vi "Insert LVClass Property Node - Tests.vi"(8 "error in (no error)":errorcluster) -> (0 "error out":errorcluster)   [LabVIEW 2017]
uses:
  myChildClass/myChildClass.lvclass
  myOtherClass.lvclass
  0cfaee32-47ef-4325-a365-739cce7879ef.vi
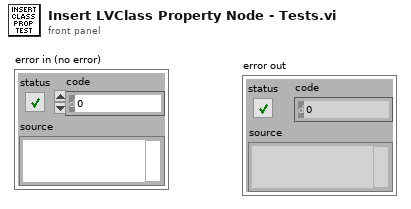
[diagram p1: front panel]
types:
  T1 = enum16{"Right Mouse Down", "Right Mouse Up", "Middle Mouse Down", "Middle Mouse Up", "Left Mouse Down", "Left Mouse Up"}
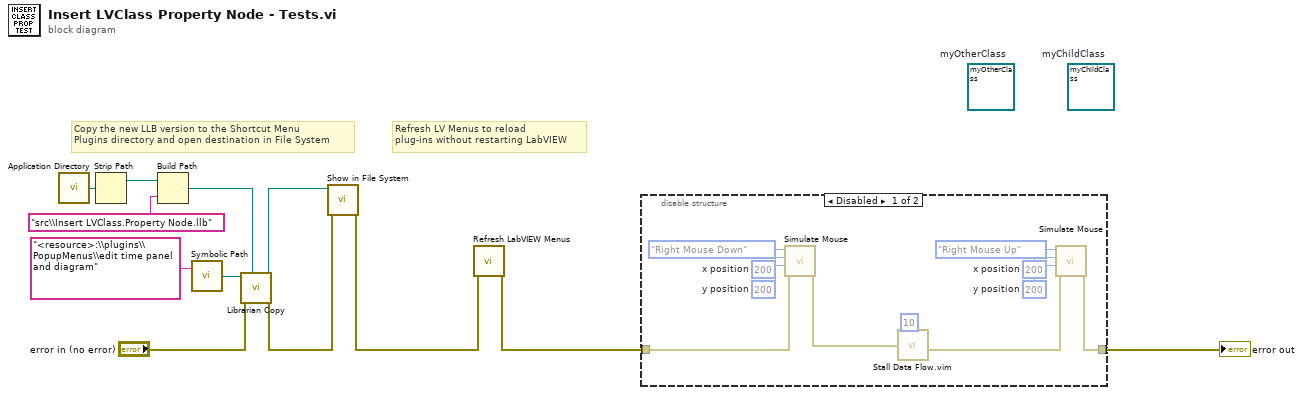
[diagram p0: block diagram]
diagram:
  (unwired) refnum<class "myOtherClass.lvclass"> refnum  # myOtherClass
  (unwired) refnum<class "myChildClass.lvclass"> refnum  # myChildClass
  # "Refresh LV Menus to reload \nplug-ins without restarting LabVIEW"
  # "Copy the new LLB version to the Shortcut Menu \nPlugins directory and open destination in File System"
  n1 = call <vilib>:"Application Directory.vi"() -> ("Application Directory"=w12:path)
  n2 = Strip Path(path=w12) -> (stripped path=w11:path)  [unwired: 1 out]
  n3 = Build Path(base path=w11, name or relative path="src\\Insert LVClass.Property Node.llb") -> (appended path=w9:path)
  n4 = call "Symbolic Path.vi"("Symbolic Path"="<resource>:\\plugins\\PopupMenus\\edit time panel and diagram" ("name or relative path")) -> ("ActualPath"=w1:path)  [unwired: 1 in]
  n5 = call <vilib>:"Librarian Copy.vi"("source"=w9, "error in (no error)"="error in (no error)", "destination"=w1) -> ("error out"=w7:errorcluster, "dup destination"=w8:path)  [unwired: 7 in]
  n6 = call <vilib>:"Show in File System.vi"("error in (no error)"=w7, "file or directory path"=w8) -> ("error out"=w6:errorcluster)  [unwired: 9 in]
  n7 = call "Refresh LabVIEW Menus.vi"("error in (no error)"=w6) -> ("error out"=w5:errorcluster)  [unwired: 10 in]
  n8 = disable-structure shown="Disabled" {
    disable-tunnel: w5 -> [w18 _]
    disable-tunnel: [w13 _] -> w3
    frame Disabled {
      w14 = 200  # x position
      w15 = 200  # y position
      w16 = 200  # x position
      w17 = 200  # y position
      n9 = call "Simulate Mouse.vi"("error in (no error)"=w18, "y position"=w17, "x position"=w16, "Action"=T1."Right Mouse Down") -> ("error out"=w21:errorcluster)  [unwired: 7 in]
      n10 = call "Stall Data Flow.vim"("value in"=w21, "milliseconds to wait"=u32 10) -> ("value out"=w20:errorcluster)  [unwired: 1 out]
      n11 = call "Simulate Mouse.vi"("error in (no error)"=w20, "y position"=w15, "x position"=w14, "Action"=T1."Right Mouse Up") -> ("error out"=w13:errorcluster)  [unwired: 7 in]
    }
    frame Enabled {
    }
  }
  "error out" <- w3
